vi "niDTS Calibration Cal IsNeeded RF Test Initialize.vi"(0 "Dut Reference":T2, 5 "SystemTechnologyCatalog":refnum<class "niDTS SystemTechnologyCatalog.lvclass">, 7 "SystemDut":refnum<class "niDTS SystemDut.lvclass">, 9 "Logger Reference":T1, 11 "error in (no error)":errorcluster) -> (4 "Template Tx Test Handle":T3, 6 "AllowAsync":bool=TRUE, 15 "error out":errorcluster)   [LabVIEW 2014, in "niDTS Utilities.lvlib"]
uses:
  niDTS Utilities.lvlib
  Includes/niDTS Calibration Cal IsNeeded RF Test INC Handle.ctl
  Objects/BASE_class/niDTS Calibration Cal IsNeeded RF Test.lvclass
  Framework/Dut/Includes/niDTS Dut INC Handle.ctl
  Framework/Dut/Objects/BASE_class/niDTS Dut.lvclass
  Framework/Logger/Includes/niDTS Logger INC Handle.ctl
  Framework/Logger/Objects/BASE_class/niDTS Logger.lvclass
  TestStand/Station/Objects/SystemTechnologyCatalog/niDTS SystemTechnologyCatalog.lvclass
  TestStand/Station/Objects/SystemDut/niDTS SystemDut.lvclass
  TestStand/niDTS TestStand.lvlib
  Framework/niDTS Framework.lvlib
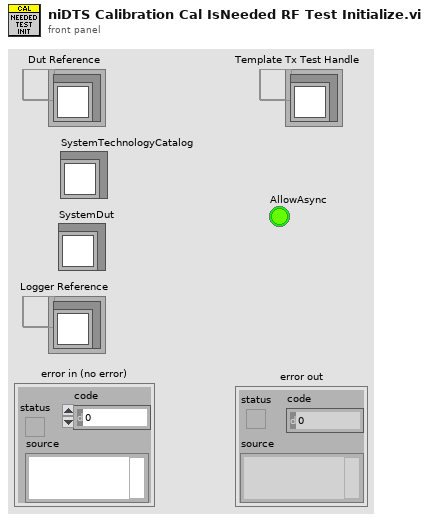
[diagram p1: front panel]
types:
  T1 = typedef "niDTS Framework.lvlib/niDTS Logger INC Handle.ctl" = refnum<data-value>
  T2 = typedef "niDTS Framework.lvlib/niDTS Dut INC Handle.ctl" = refnum<data-value>
  T3 = typedef "niDTS Utilities.lvlib/niDTS Calibration Cal IsNeeded RF Test INC Handle.ctl" = refnum<data-value>
  T4 = typedef "niDTS TestStand.lvlib/niDTS TestStep INC Handle.ctl" = refnum<data-value>
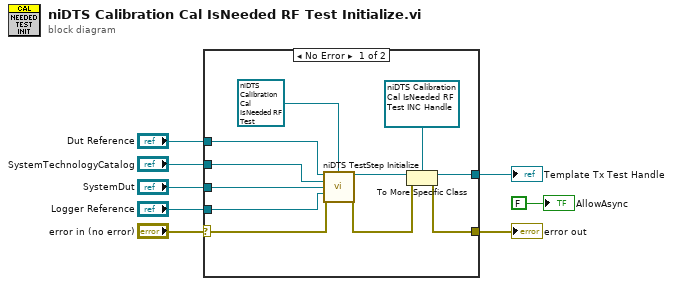
[diagram p0: block diagram]
diagram:
  n1 = case shown="No Error" "error in (no error)" {
    selector: "error in (no error)" -> [w13 w20]
    tunnel: [w19 w20] -> w8
    tunnel: [w18 _] -> w6
    tunnel: "Logger Reference" -> [w12 _]
    tunnel: "SystemDut" -> [w11 _]
    tunnel: "SystemTechnologyCatalog" -> [w10 _]
    tunnel: "Dut Reference" -> [w9 _]
    frame No Error {
      n2 = call "niDTS TestStep Initialize.vi"("Dut Handle"=w9, "Test Type"=refnum<class "niDTS Calibration Cal IsNeeded RF Test.lvclass"> refnum ("Template.lvlib:Template Tx Test.lvclass"), "SystemTechnologyCatalog"=w10, "SystemDut"=w11, "Logger Reference"=w12, "error in (no error)"=w13) -> ("Test Handle out"=w15:T4, "error out"=w14:errorcluster)  [unwired: 8 in]
      n3 = To More Specific Class(target class=T3 refnum ("Template Tx Test Handle"), reference=w15, error in=w14) -> (specific class reference=w18:T3, error out=w19:errorcluster)
    }
    frame Error {
    }
  }
  "error out" <- w8
  "Template Tx Test Handle" <- w6
  "AllowAsync" <- FALSE ("AllowAsync")
